vi "Simple Reader.vi"(8 "error in (no error)":errorcluster, 11 "IPS120 in":refnum<class "IPS120.lvclass">) -> (0 "error out":errorcluster, 2 "Signals":dbl[](array[numeric]), 3 "IPS120 out":refnum<class "IPS120.lvclass">)   [LabVIEW 2025, in "IPS120.lvclass"]
uses:
  IPS120.lvclass
  C:/GitHub/NHMFL_Core/Libraries/Instruments/VISA Instrument/VISA Instrument.lvclass
  VISA Instrument/VISA Instrument.lvclass/VISA Instrument.ctl
  VISA Instrument/Read VISA resource.vi
  VISA Instrument/Write VISA resource.vi
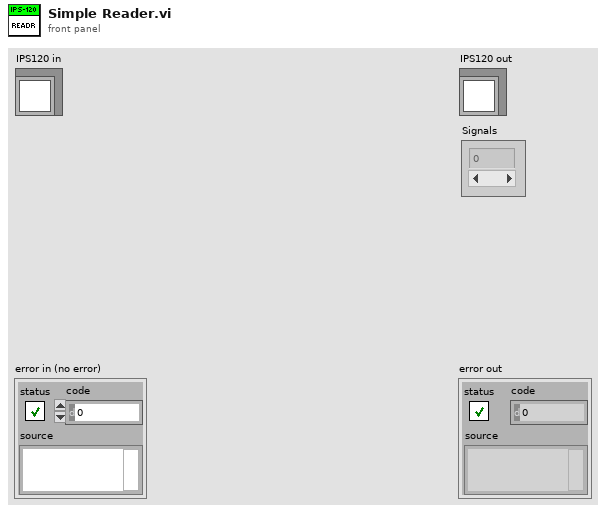
[diagram p1: front panel]
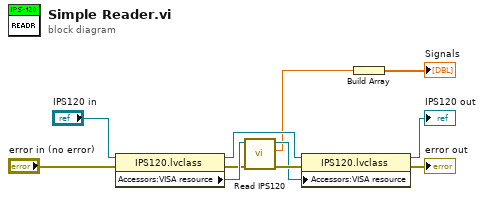
[diagram p0: block diagram]
diagram:
  n1 = property class="IPS120.lvclass"(reference="IPS120 in", error in="error in (no error)") -> (reference out=w10:refnum<class "IPS120.lvclass">, error out=w5:errorcluster, "Accessors:VISA resource"=w6:refnum<visa-resource-name>)
  n2 = call "Read IPS120.vi"("error in (no error)"=w5, "VISA resource name"=w6) -> ("error out"=w4:errorcluster, "Value"=w2:dbl, "VISA resource name out"=w3:refnum<visa-resource-name>)  [unwired: 5 in, 2 out]
  n3 = property class="IPS120.lvclass"(reference=w10, error in=w4, "Accessors:VISA resource"=w3) -> (reference out=→"IPS120 out":refnum<class "IPS120.lvclass">, error out=→"error out":errorcluster)
  n4 = Build Array(w2) -> (→"Signals":dbl[])
